vi "CalcTunJunctionRVandError.vi"(5 "Rp":dbl format="%#_13g", 7 "Rl":dbl format="%#_13g", 8 "Source Voltage (V)":dbl format="%#_13g", 9 "Sample Current StDev (A)":dbl format="%#_13g", 10 "Sample Current Theta (degrees)":dbl format="%#_13g", 11 "Sample Current R (A)":dbl format="%#_13g") -> (0 "Sample Resistance StDev (Ohms)":dbl, 1 "Sample Resistance (Ohms)":dbl, 2 "Sample Voltage StDev (V)":dbl, 3 "Sample Voltage (V)":dbl)   [LabVIEW 2016]
panel:
  # "This VI assumes use of the swithc box to measure the resistance of a high resistance sample\n(usually some form of tunnel junction, but could just be a large resistor). It treats the sample \nas a parallel combination of a resistor and capacitor to account for the measurable reactance of the \nthe parasitic ground capacitatance."
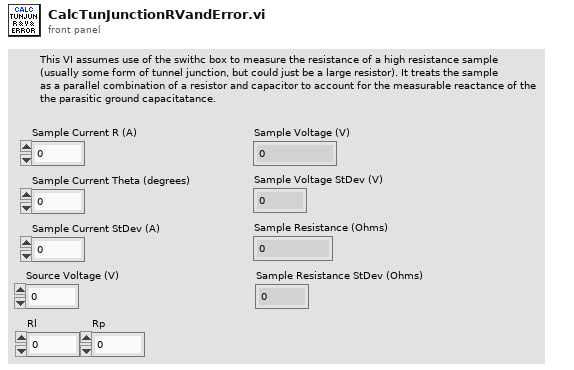
[diagram p1: front panel]
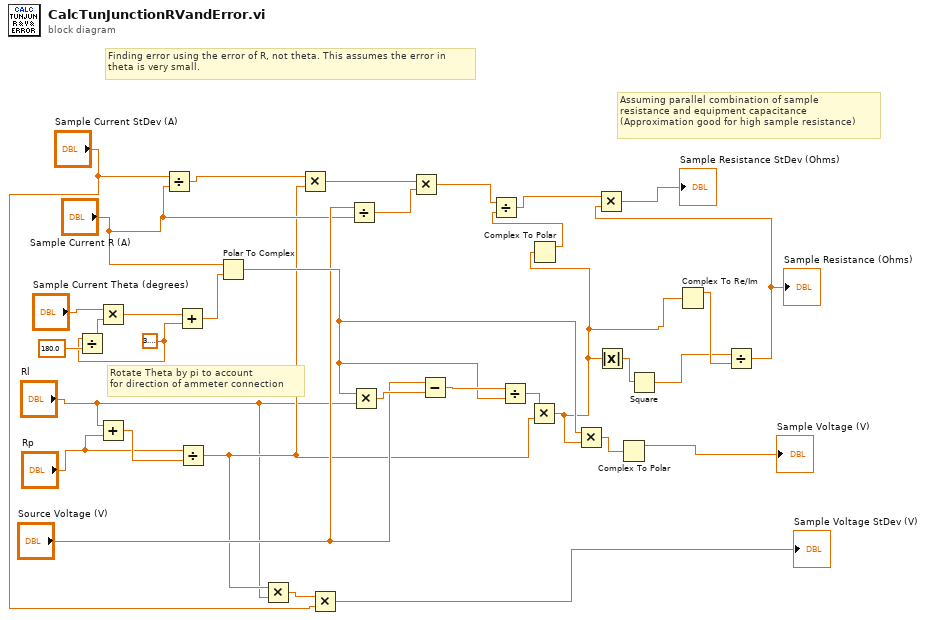
[diagram p0: block diagram]
diagram:
  w2 = 3.141592653589793
  # "Finding error using the error of R, not theta. This assumes the error in \ntheta is very small."
  # "Assuming parallel combination of sample\nresistance and equipment capacitance\n(Approximation good for high sample resistance)"
  # "Rotate Theta by pi to account\nfor direction of ammeter connection"
  n1 = Divide(x=w2, y=180.0) -> (x/y=w1:dbl)
  n2 = Multiply(x="Sample Current Theta (degrees)", y=w1) -> (x*y=w4:dbl)
  n3 = Add(x="Rl", y="Rp") -> (x+y=w31:dbl)
  n4 = Divide(x="Sample Current StDev (A)", y="Sample Current R (A)") -> (x/y=w25:dbl)
  n5 = Add(x=w4, y=w2) -> (x+y=w27:dbl)
  n6 = Divide(x="Rp", y=w31) -> (x/y=w10:dbl)
  n7 = Polar To Complex(1:w27, 2:"Sample Current R (A)") -> (0:w28:cdb)
  n8 = Multiply(x=w10, y="Rl") -> (x*y=w8:dbl)
  n9 = Multiply(x=w25, y=w10) -> (x*y=w21:dbl)
  n10 = Multiply(x=w8, y="Sample Current StDev (A)") -> (x*y=→"Sample Voltage StDev (V)":dbl)
  n11 = Divide(x="Source Voltage (V)", y="Sample Current R (A)") -> (x/y=w22:dbl)
  n12 = Multiply(x=w28, y="Rl") -> (x*y=w33:cdb)
  n13 = Multiply(x=w21, y=w22) -> (x*y=w20:dbl)
  n14 = Subtract(x="Source Voltage (V)", y=w33) -> (x-y=w32:cdb)
  n15 = Divide(x=w32, y=w28) -> (x/y=w29:cdb)
  n16 = Multiply(x=w29, y=w10) -> (x*y=w16:cdb)
  n17 = Complex To Polar(r * e^(i*theta)=w16) -> (r=w19:dbl)  [unwired: 1 out]
  n18 = Divide(x=w20, y=w19) -> (x/y=w18:dbl)
  n19 = Multiply(x=w28, y=w16) -> (x*y=w12:cdb)
  n20 = Absolute Value(x=w16) -> (abs(x)=w15:dbl)
  n21 = Complex To Polar(r * e^(i*theta)=w12) -> (r=→"Sample Voltage (V)":dbl)  [unwired: 1 out]
  n22 = Square(x=w15) -> (x^2=w14:dbl)
  n23 = Complex To Re/Im(x + iy=w16) -> (x=w26:dbl)  [unwired: 1 out]
  n24 = Divide(x=w14, y=w26) -> (x/y=w17:dbl)
  "Sample Resistance (Ohms)" <- w17
  n25 = Multiply(x=w18, y=w17) -> (x*y=→"Sample Resistance StDev (Ohms)":dbl)
